vi "Write.vi"(8 "error in (no error)":errorcluster, 10 "write buffer":string, 11 "Serial Logging Decorator In":refnum<class "Serial Logging Decorator.lvclass">) -> (0 "error out":errorcluster, 2 "return count":u32, 3 "Serial Logging Decorator Out":refnum<class "Serial Logging Decorator.lvclass">)   [LabVIEW 2020, in "Serial Logging Decorator.lvclass"]
uses:
  Serial Logging Decorator.lvclass
  Serial Logging Decorator.lvclass/Serial Logging Decorator.ctl
  Log/Log.lvclass
  Serial/Serial.lvclass/Serial.lvclass
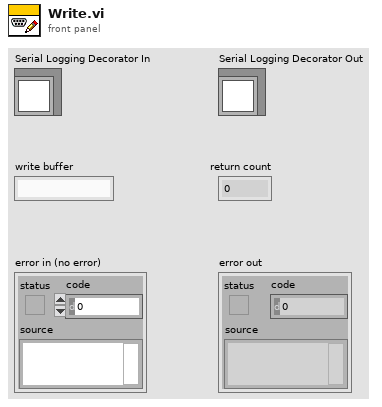
[diagram p1: front panel]
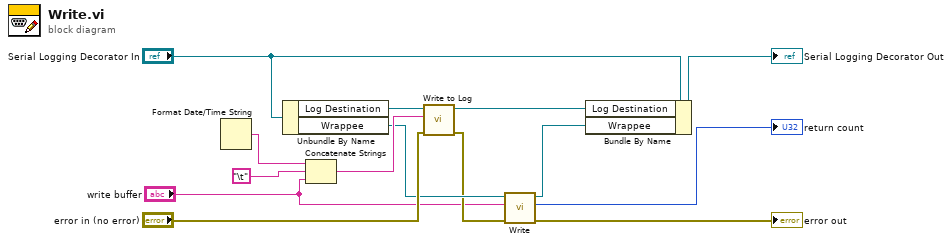
[diagram p0: block diagram]
diagram:
  n1 = Format Date/Time String() -> (date/time string=w9:string)  [unwired: 3 in]
  n2 = Unbundle By Name("Serial Logging Decorator In") -> ("Log Destination"=w13:refnum<class "Log.lvclass">, "Wrappee"=w6:refnum<class "Serial.lvclass">)
  n3 = Concatenate Strings(w9, "\t" ("string"), "write buffer") -> (w7:string)
  n4 = call-dynamic "Write to Log.vi"("error in (no error)"="error in (no error)", "Text to Write"=w7, "Log in"=w13) -> ("error out"=w5:errorcluster, "Log out"=w11:refnum<class "Log.lvclass">)  [unwired: 7 in]
  n5 = call-dynamic "Write.vi"("error in (no error)"=w5, "write buffer"="write buffer", "Serial in"=w6) -> ("error out"=→"error out":errorcluster, "return count"=→"return count":u32, "Serial out"=w3:refnum<class "Serial.lvclass">)  [unwired: 6 in]
  n6 = Bundle By Name(cluster="Serial Logging Decorator In", "Log Destination"=w11, "Wrappee"=w3) -> (→"Serial Logging Decorator Out":refnum<class "Serial Logging Decorator.lvclass">)
